vi "init.vi"(11 "ttm_poller_panel.vi.lvclass":refnum<class "ttmServer.lvclass">) -> (3 "output cluster":refnum<class "ttmServer.lvclass">)   [LabVIEW 2011, in "ttmServer.lvclass"]
uses:
  ttmServer.lvclass
  ttmServer.lvclass/ttmServer.ctl
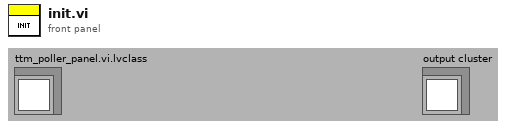
[diagram p1: front panel]
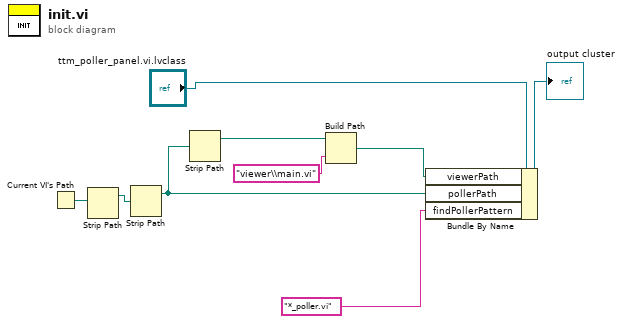
[diagram p0: block diagram]
diagram:
  n1 = Current VI's Path() -> (path=w9:path)
  n2 = Strip Path(path=w9) -> (stripped path=w8:path)  [unwired: 1 out]
  n3 = Strip Path(path=w8) -> (stripped path=w3:path)  [unwired: 1 out]
  n4 = Strip Path(path=w3) -> (stripped path=w1:path)  [unwired: 1 out]
  n5 = Build Path(base path=w1, name or relative path="viewer\\main.vi") -> (appended path=w2:path)
  n6 = Bundle By Name(cluster="ttm_poller_panel.vi.lvclass", "viewerPath"=w2, "pollerPath"=w3, "findPollerPattern"="*_poller.vi") -> (→"output cluster":refnum<class "ttmServer.lvclass">)
